vi "StringMeasure.vi"(5 "EndTime":timestamp, 7 "StartTime":timestamp, 8 "error in":errorcluster, 11 "StringMeasure":refnum<class "StringMeasure.lvclass">) -> (0 "error out":errorcluster, 3 "Passed":bool)   [LabVIEW 2020]
uses:
  <vilib>/Averna/ProligentResultProcessor/ProligentResultProcessor.lvlibp/Measure/StringMeasure/StringMeasure.lvclass
  C:/Program Files (x86)/National Instruments/LabVIEW 2020/vi.lib/Averna/ProligentResultProcessor/ProligentResultProcessor.lvlibp/Measure/Measure/Measure.lvclass
  <vilib>/Averna/ProligentResultProcessor/ProligentResultProcessor.lvlibp/Measure/StringMeasureLimit/StringMeasureLimit.lvclass
  C:/Program Files (x86)/National Instruments/LabVIEW 2020/vi.lib/Averna/ProligentResultProcessor/ProligentResultProcessor.lvlibp/Measure/MeasureLimit/MeasureLimit.lvclass
  <vilib>/Averna/ProligentResultProcessor/ProligentResultProcessor.lvlibp/Measure/Measure/SetStartDate.vi
  <vilib>/Averna/ProligentResultProcessor/ProligentResultProcessor.lvlibp/Measure/Measure/SetMeasureExecutionStatus.vi
  <vilib>/Averna/ProligentResultProcessor/ProligentResultProcessor.lvlibp/Measure/StringMeasure/SetValue.vi
  <vilib>/Averna/ProligentResultProcessor/ProligentResultProcessor.lvlibp/Measure/Measure/SetComments.vi
  <vilib>/Averna/ProligentResultProcessor/ProligentResultProcessor.lvlibp/Measure/Measure/SetMeasureId.vi
  <vilib>/Averna/ProligentResultProcessor/ProligentResultProcessor.lvlibp/Measure/Measure/GetStartDate.vi
  <vilib>/Averna/ProligentResultProcessor/ProligentResultProcessor.lvlibp/Measure/Measure/GetMeasureExecutionStatus.vi
  <vilib>/Averna/ProligentResultProcessor/ProligentResultProcessor.lvlibp/Measure/StringMeasure/GetValue.vi
  <vilib>/Averna/ProligentResultProcessor/ProligentResultProcessor.lvlibp/Measure/Measure/GetComments.vi
  <vilib>/Averna/ProligentResultProcessor/ProligentResultProcessor.lvlibp/Measure/Measure/GetMeasureId.vi
  <vilib>/Averna/ProligentResultProcessor/ProligentResultProcessor.lvlibp/Measure/Measure/GetLimit.vi
  <vilib>/Averna/ProligentResultProcessor/ProligentResultProcessor.lvlibp/Measure/StringMeasureLimit/SetComparison.vi
  <vilib>/Averna/ProligentResultProcessor/ProligentResultProcessor.lvlibp/Measure/StringMeasureLimit/GetComparison.vi
  <vilib>/Averna/ProligentResultProcessor/ProligentResultProcessor.lvlibp/Measure/MeasureLimit/GetLimitExpression.vi
  <vilib>/Averna/ProligentResultProcessor/ProligentResultProcessor.lvlibp/Measure/MeasureLimit/GetCustomData.vi
  <vilib>/Averna/ProligentResultProcessor/ProligentResultProcessor.lvlibp/Measure/Measure/GetCharacteristics.vi
  <vilib>/Averna/ProligentResultProcessor/ProligentResultProcessor.lvlibp/Measure/Measure/GetFailureReferences.vi
  <vilib>/Averna/ProligentResultProcessor/ProligentResultProcessor.lvlibp/Measure/Measure/GetCustomData.vi
  <vilib>/Averna/ProligentResultProcessor/ProligentResultProcessor.lvlibp/Measure/MeasureLimit/MeasureLimit.lvclass
  <vilib>/Averna/ProligentResultProcessor/ProligentResultProcessor.lvlibp/Model/CustomData/CustomData.lvclass
  <vilib>/Averna/ProligentResultProcessor/ProligentResultProcessor.lvlibp/Model/Characteristic/Characteristic.lvclass
  <vilib>/Averna/ProligentResultProcessor/ProligentResultProcessor.lvlibp/Failure/FailureReference/FailureReference.lvclass
  <vilib>/Averna/ProligentResultProcessor/ProligentResultProcessor.lvlibp/Measure/Measure/Measure.lvclass
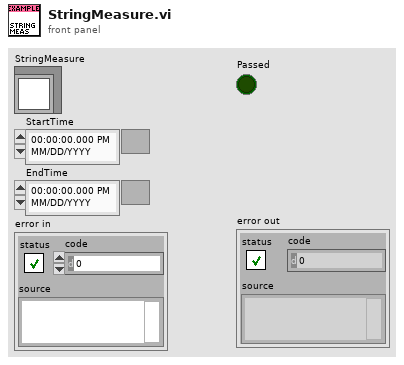
[diagram p1: front panel]
types:
  T1 = enum16{"PASS", "FAIL", "NOT_COMPLETED", "ABORTED"}
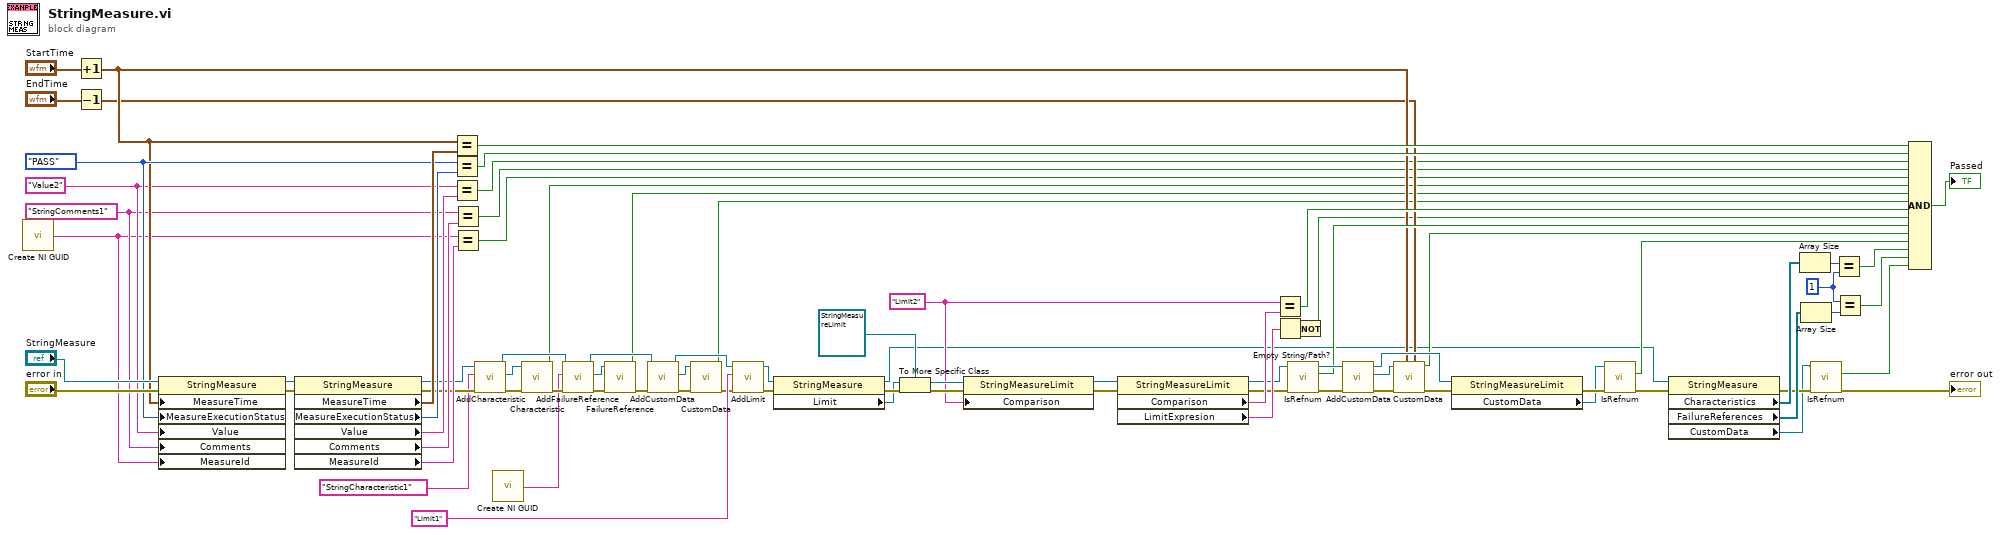
[diagram p0: block diagram]
diagram:
  w30 = 1
  w38 = "StringComments1"
  w41 = "Limit2"
  w43 = "Value2"
  w72 = T1."PASS" ("ProcessRunStatus")
  n1 = call <vilib>:"Create NI GUID.vi"() -> ("NI GUID"=w35:string)
  n2 = Increment(x="StartTime") -> (x+1=w46:timestamp)
  n3 = Decrement(x="EndTime") -> (x-1=w45:timestamp)
  n4 = property class="StringMeasure"(reference="StringMeasure", error in="error in", "MeasureTime"=w46, "MeasureExecutionStatus"=w72, "Value"=w43, "Comments"=w38, "MeasureId"=w35) -> (reference out=w82:refnum<class "StringMeasure.lvclass">, error out=w81:errorcluster)
  n5 = property class="StringMeasure"(reference=w82, error in=w81) -> (reference out=w9:refnum<class "StringMeasure.lvclass">, error out=w7:errorcluster, "MeasureTime"=w80:timestamp, "MeasureExecutionStatus"=w79:T1, "Value"=w78:string, "Comments"=w37:string, "MeasureId"=w36:string)
  n6 = Equal?(x=w46, y=w80) -> (x = y?=w77:bool)
  n7 = Equal?(x=w72, y=w79) -> (x = y?=w76:bool)
  n8 = Equal?(x=w43, y=w78) -> (x = y?=w39:bool)
  n9 = Equal?(x=w38, y=w37) -> (x = y?=w34:bool)
  n10 = Equal?(x=w35, y=w36) -> (x = y?=w33:bool)
  n11 = call <vilib>:"AddCharacteristic.vi"("error in (no error)"=w7, "FullName"="StringCharacteristic1", "Measure in"=w9) -> ("error out"=w19:errorcluster, "Characteristic"=w18:refnum<class "Characteristic.lvclass">, "Measure out"=w16:refnum<class "StringMeasure.lvclass">)  [unwired: 6 in]
  n12 = call <vilib>:"Create NI GUID.vi"() -> ("NI GUID"=w1:string)
  n13 = call "Characteristic.vi"("error in (no error)"=w19, "Characteristic in"=w18) -> ("error out"=w17:errorcluster, "Passed"=w5:bool)  [unwired: 8 in]
  n14 = call <vilib>:"AddFailureReference.vi"("error in (no error)"=w17, "Id"=w1, "Measure in"=w16) -> ("error out"=w11:errorcluster, "FailureReference"=w10:refnum<class "FailureReference.lvclass">, "Measure out"=w13:refnum<class "StringMeasure.lvclass">)  [unwired: 6 in]
  n15 = call "FailureReference.vi"("error in"=w11, "FailureReference"=w10) -> ("error out"=w15:errorcluster, "Passed"=w4:bool)  [unwired: 8 in]
  n16 = call <vilib>:"AddCustomData.vi"("error in (no error)"=w15, "Measure in"=w13) -> ("error out"=w14:errorcluster, "CustomData"=w12:refnum<class "CustomData.lvclass">, "Measure out"=w8:refnum<class "StringMeasure.lvclass">)  [unwired: 7 in]
  n17 = call "CustomData.vi"("error in"=w14, "CustomData"=w12) -> ("error out"=w6:errorcluster, "Passed"=w3:bool)  [unwired: 8 in]
  n18 = call <vilib>:"AddLimit.vi"("error in"=w6, "Comparison"="Limit1", "StringMeasure in"=w8) -> ("error out"=w65:errorcluster, "StringMeasure out"=w71:refnum<class "StringMeasure.lvclass">)  [unwired: 6 in, 1 out]
  n19 = property class="StringMeasure"(reference=w71, error in=w65) -> (reference out=w26:refnum<class "StringMeasure.lvclass">, error out=w70:errorcluster, "Limit"=w66:refnum<class "MeasureLimit.lvclass">)
  n20 = To More Specific Class(target class=refnum<class "StringMeasureLimit.lvclass"> refnum ("ProligentResultProcessor:StringMeasureLimit"), reference=w66, error in=w70) -> (specific class reference=w67:refnum<class "StringMeasureLimit.lvclass">, error out=w69:errorcluster)
  n21 = property class="StringMeasureLimit"(reference=w67, error in=w69, "Comparison"=w41) -> (reference out=w64:refnum<class "StringMeasureLimit.lvclass">, error out=w63:errorcluster)
  n22 = property class="StringMeasureLimit"(reference=w64, error in=w63) -> (reference out=w53:refnum<class "StringMeasureLimit.lvclass">, error out=w58:errorcluster, "Comparison"=w62:string, "LimitExpresion"=w61:string)
  n23 = Equal?(x=w41, y=w62) -> (x = y?=w60:bool)
  n24 = Empty String/Path?(string/path=w61) -> (empty?=w59:bool)
  n25 = call <vilib>:"IsRefnum.vi"("error in"=w58, "MeasureLimit in"=w53) -> ("error out"=w54:errorcluster, "IsRefnum"=w51:bool, "MeasureLimit out"=w52:refnum<class "StringMeasureLimit.lvclass">)  [unwired: 7 in]
  n26 = Not(x=w59) -> (.not. x?=w40:bool)
  n27 = call <vilib>:"AddCustomData.vi"("error in"=w54, "MeasureLimit in"=w52) -> ("error out"=w49:errorcluster, "CustomData"=w47:refnum<class "CustomData.lvclass">, "MeasureLimit out"=w50:refnum<class "StringMeasureLimit.lvclass">)  [unwired: 7 in]
  n28 = call "CustomData.vi"("EndTime"=w45, "StartTime"=w46, "error in"=w49, "CustomData"=w47) -> ("error out"=w48:errorcluster, "Passed"=w44:bool)  [unwired: 6 in]
  n29 = property class="StringMeasureLimit"(reference=w50, error in=w48) -> (error out=w57:errorcluster, "CustomData"=w56:refnum<class "CustomData.lvclass">)  [unwired: 1 out]
  n30 = call <vilib>:"IsRefnum.vi"("error in"=w57, "CustomDataType in"=w56) -> ("error out"=w23:errorcluster, "IsRefnum"=w55:bool)  [unwired: 7 in, 1 out]
  n31 = property class="StringMeasure"(reference=w26, error in=w23) -> (error out=w22:errorcluster, "Characteristics"=w25:refnum<class "Characteristic.lvclass">[], "FailureReferences"=w24:refnum<class "FailureReference.lvclass">[], "CustomData"=w20:refnum<class "CustomData.lvclass">)  [unwired: 1 out]
  n32 = Array Size(array=w25) -> (size(s)=w32:i32)
  n33 = Array Size(array=w24) -> (size(s)=w31:i32)
  n34 = call <vilib>:"IsRefnum.vi"("error in"=w22, "CustomDataType in"=w20) -> ("error out"=→"error out":errorcluster, "IsRefnum"=w29:bool)  [unwired: 7 in, 1 out]
  n35 = Equal?(x=w32, y=w30) -> (x = y?=w27:bool)
  n36 = Equal?(x=w30, y=w31) -> (x = y?=w28:bool)
  n37 = Compound Arithmetic op=AND(w77, w76, w39, w34, w33, w5, w4, w3, w60, w40, w51, w44, w55, w27, w28, w29) -> (→"Passed":bool)
